vi "import outnames.vi"(11 "units":string(combo)) -> (3 "String Array From File":string[][](array[string]))   [LabVIEW 2017]
uses:
  <vilib>/Utility/file.llb/Read Delimited Spreadsheet (string).vi
panel:
  in  "Search String":string
  out "Check Array":dbl[](array[numeric])
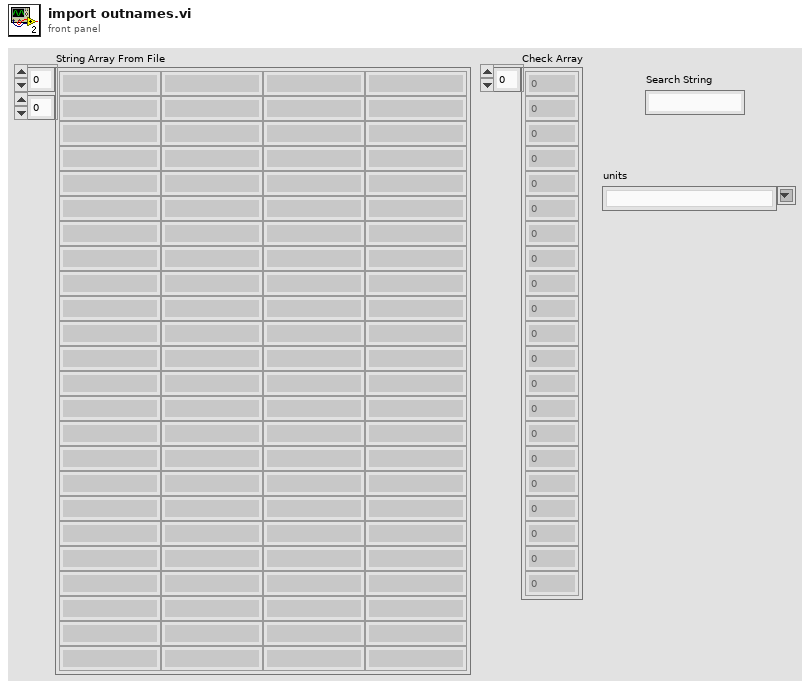
[diagram p1: front panel]
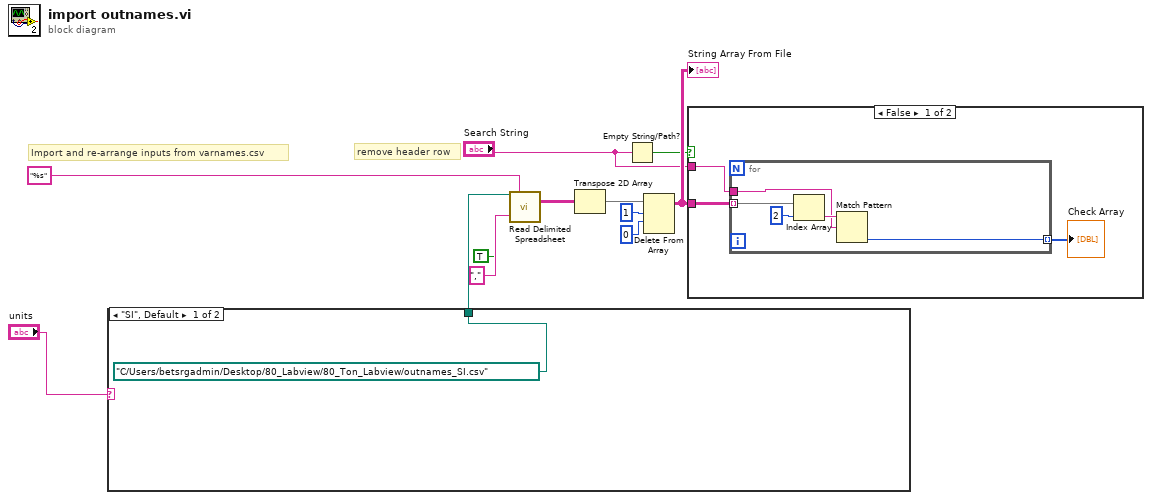
[diagram p0: block diagram]
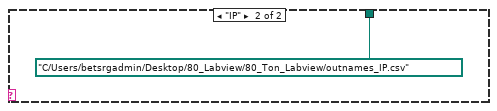
[diagram p2: hidden frame]
diagram:
  # "remove header row"
  # "Import and re-arrange inputs from varnames.csv"
  n1 = case shown="\"SI\", Default" "units" {
    tunnel: [path "C:/Users/betsrgadmin/Desktop/80_Labview/80_Ton_Labview/outnames_SI.csv" path "C:/Users/betsrgadmin/Desktop/80_Labview/80_Ton_Labview/outnames_IP.csv"] -> w10
    frame "SI", Default {
    }
    frame "IP" {
    }
  }
  n2 = call-poly <vilib>:"Read Delimited Spreadsheet.vi"("file path (dialog if empty)"=w10, "format (%s)"="%s", "transpose? (F)"=TRUE, "delimiter (\\t)"=",") -> ("all rows"=w8:string[][])  [unwired: 6 in, 5 out]
  n3 = Transpose 2D Array(2D array=w8) -> (transposed array=w7:string[][])
  n4 = Empty String/Path?(string/path="Search String") -> (empty?=w3:bool)
  n5 = Delete From Array(array=w7, length=1, index (row)=0) -> (array with subset deleted=w4:string[][])  [unwired: 1 in, 1 out]
  "String Array From File" <- w4
  n6 = case shown="False" w3 {
    tunnel: w4 -> [w16 _]
    tunnel: "Search String" -> [w15 _]
    frame False {
      n7 = for {
        tunnel: w16 -> [w22] mode=indexing
        tunnel: [w20] -> w17 mode=indexing
        tunnel: w15 -> [w18]
        n8 = Index Array(array=w22, index=2) -> (element=w21:string)
        n9 = Match Pattern(string=w21, regular expression=w18) -> (offset past match=w20:i32)  [unwired: 1 in, 3 out]
      }
      "Check Array" <- w17
    }
    frame True {
    }
  }
